vi "Draw Lines First.vi"(8 "error in (no error)":errorcluster, 11 "Refnum in":T1) -> (0 "error out":errorcluster, 3 "Refnum out":T1)   [LabVIEW 2019]
doc: "This VI draws a point at the origin to register the lines group. This ensures that the line layer is the bottom-most layer."
uses:
  <vilib>/vision/Image Controls.llb/IMAQ Image.ctl
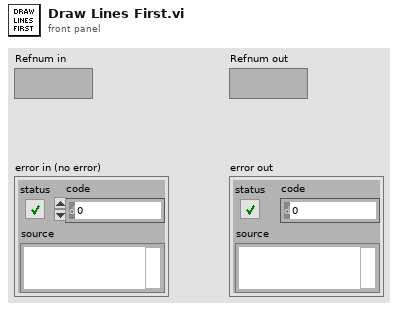
[diagram p1: front panel]
types:
  T1 = typedef "IMAQ Image.ctl" = refnum<image>
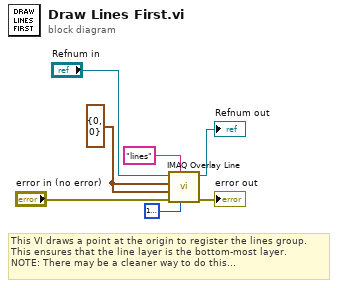
[diagram p0: block diagram]
diagram:
  w2 = cluster{"X":i32, "Y":i32} {"X"=0, "Y"=0} ("Start Point")
  # "This VI draws a point at the origin to register the lines group.\nThis ensures that the line layer is the bottom-most layer.\nNOTE: There may be a cleaner way to do this..."
  n1 = call "IMAQ Overlay Line"("Color"=u32 16777216, "Group"="lines", "error in (no error)"="error in (no error)", "End Point"=w2, "Start Point"=w2, "Image"="Refnum in") -> ("error out"=→"error out":errorcluster, "Image Out"=→"Refnum out":T1)  [unwired: 4 in]
